vi "Read Datagram.vi"(8 "error in (no error)":errorcluster, 10 "Transfer Group Rx parameters":T1={"Transfers Rx"=[], "max size"=548} {"max size" format="%d bytes"; "Transfers Rx"."source address" format="%d ms"; "Transfers Rx"."timeout" format="%d bytes"}, 11 "UDP Transceiver in":refnum<class "UDP Transceiver.lvclass">) -> (0 "error out":errorcluster, 1 "data":string, 2 "Transfer index":i32, 3 "UDP Transceiver out":refnum<class "UDP Transceiver.lvclass">)   [LabVIEW 2017, in "UDP.lvlib" / "UDP Transceiver.lvclass"]
uses:
  UDP Transceiver.lvclass
  Transfer Group Rx Parameters.ctl
  Transfer Rx Parameters.ctl
  UDP Transceiver.lvclass/UDP Transceiver.ctl
  UDP Unknown Datagram Error.vi
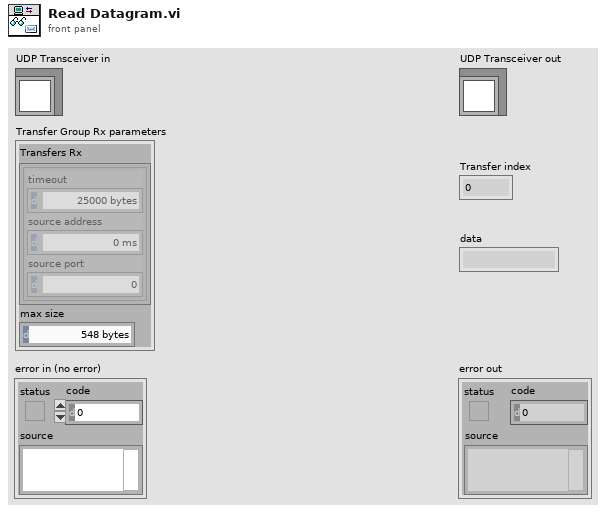
[diagram p1: front panel]
types:
  T1 = typedef "UDP.lvlib/UDP Transceiver.lvclass/Transfer Group Rx Parameters.ctl" = cluster{"Transfers Rx":T2[], "max size":i32}
  T2 = typedef "UDP.lvlib/UDP Transceiver.lvclass/Transfer Rx Parameters.ctl" = cluster{"timeout":i32, "source address":u32, "source port":u16}
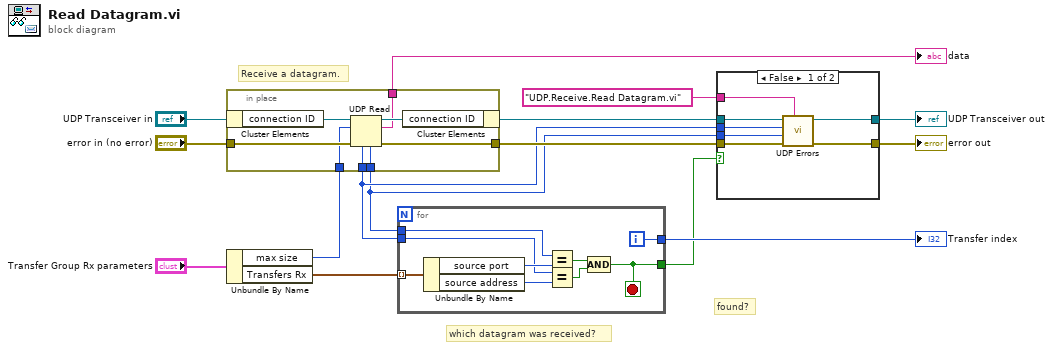
[diagram p0: block diagram]
diagram:
  # "found?"
  # "Receive a datagram."
  # "which datagram was received?"
  n1 = Unbundle By Name("Transfer Group Rx parameters") -> ("max size"=w14:i32, "Transfers Rx"=w13:T2[])
  n2 = in-place {
    in-place-border: "error in (no error)" -> [w23]
    in-place-border: [w21] -> w12
    in-place-border: [w19] -> w10
    in-place-border: [w18] -> w9
    in-place-border: w14 -> [w17]
    in-place-border: [w16] -> w7
    n3 = in-place-cluster #1("UDP Transceiver in") -> ("connection ID"=w20:refnum<k16>)
    n4 = UDP Read(connection ID=w20, max size (548)=w17, 8:w23) -> (data out=w16:string, error out=w21:errorcluster, 3:w22:refnum<k16>, 4:w18:u16, 6:w19:u32)  [unwired: 1 in]
    n5 = in-place-cluster #1("connection ID"=w22) -> (w11:refnum<class "UDP Transceiver.lvclass">)
  }
  "data" <- w7
  n6 = for {
    tunnel: w13 -> [w32] mode=indexing
    tunnel: w10 -> [w29]
    tunnel: w9 -> [w28]
    tunnel: [w25] -> w8
    tunnel: [w24] -> w1
    i -> [w25]
    stop <- w24 stop-if-true
    n7 = Unbundle By Name(w32) -> ("source port"=w30:u16, "source address"=w31:u32)
    n8 = Equal?(x=w28, y=w30) -> (x = y?=w26:bool)
    n9 = Equal?(x=w29, y=w31) -> (x = y?=w27:bool)
    n10 = Compound Arithmetic op=AND(w26, w27) -> (w24:bool)
  }
  "Transfer index" <- w8
  n11 = case shown="False" w1 {
    tunnel: w12 -> [w38 w40]
    tunnel: w11 -> [w39 w41]
    tunnel: [w37 w41] -> w3
    tunnel: [w36 w40] -> w2
    tunnel: w10 -> [w35 _]
    tunnel: w9 -> [w34 _]
    tunnel: "UDP.Receive.Read Datagram.vi" ("source vi name") -> [w33 _]
    frame False {
      n12 = call-poly "UDP Errors.vi"("source vi name"=w33, "error in (no error)"=w38, "source port"=w34, "source address"=w35, "UDP in"=w39) -> ("error out"=w36:errorcluster, "UDP out"=w37:refnum<class "UDP Transceiver.lvclass">)  [unwired: 5 in]
    }
    frame True {
    }
  }
  "error out" <- w2
  "UDP Transceiver out" <- w3
